vi "Drive Train Global.vi"() -> ()   [LabVIEW 2018]
panel:
  in  "Robot Stopped?":bool=TRUE
  in  "Reset Field Position":bool
  in  "Wheel Angle Offsets Practice Bot":T1={"FrontLeft"=-142.0, "FrontRight"=107.85, "BackLeft"=-87.1, "BackRight"=69.4}
  in  "Angle Locking to":dbl=630.0
  in  "Angle to Lock To":dbl=270.0
  out "Lock to Angle":bool
  out "Robot Centric":bool
  in  "Don't Turn While Translate PID Gains":T2 {"derivative time (Td, min)" format="%.3f"; "integral time (Ti, min)" format="%.3f"; "proportional gain (Kc)" format="%.3f"}
  in  "Zero Yaw":bool
  in  "Wheel Angle Offsets":T1={"FrontLeft"=135.0, "FrontRight"=-169.4, "BackLeft"=-64.0, "BackRight"=-40.1}
  out "Wheel Angles":T1={"FrontLeft"=-0.07255429144282743, "FrontRight"=0.13487537853610831, "BackLeft"=-0.06803657905170724, "BackRight"=-0.04791306754956537}
  in  "Rot. Point Y":dbl
  in  "Rot. Point X":dbl
  in  "Wheel Turn PID Values":T3={"Front Left"={"P Value"=0.014, "I Value"=0.0, "D Value"=0.0}, "Front Right"={"P Value"=0.014, "I Value"=0.0, "D Value"=0.0}, "Back Left"={"P Value"=0.014, "I Value"=0.0, "D Value"=0.0}, "Back Right"={"P Value"=0.014, "I Value"=0.0, "D Value"=0.0}}
  in  "Z Command":dbl
  in  "Y Command":dbl=-0.0
  out "Gyro Information":T4={"Rollover"=0.0, "Yaw"=-1.63, "Cont Yaw"=-1.63}
  in  "X Command":dbl=-0.01165823673846645
  in  "Current State":enum16{"Reached Position", "Going to Position"}(ring)
  in  "Current Mode":T5(ring)=enum."Field Oriented"
  out "Extra Info":bool
  out "Velocity":cluster{"X":dbl, "Y":dbl}
  out "Position":cluster{"X":dbl, "Y":dbl}={"X"=0.31095361119092635, "Y"=-0.2016841928455702}
  out "Wheel Drive Encoders":cluster{"Rates":dbl[], "Distances":dbl[]}={"Rates"=[0.0, 0.0, 0.0, -0.0], "Distances"=[0.9954750000000001, -0.01917175, -0.287145, -0.0]}
  # "X Command is spin"
  # "Z is X"
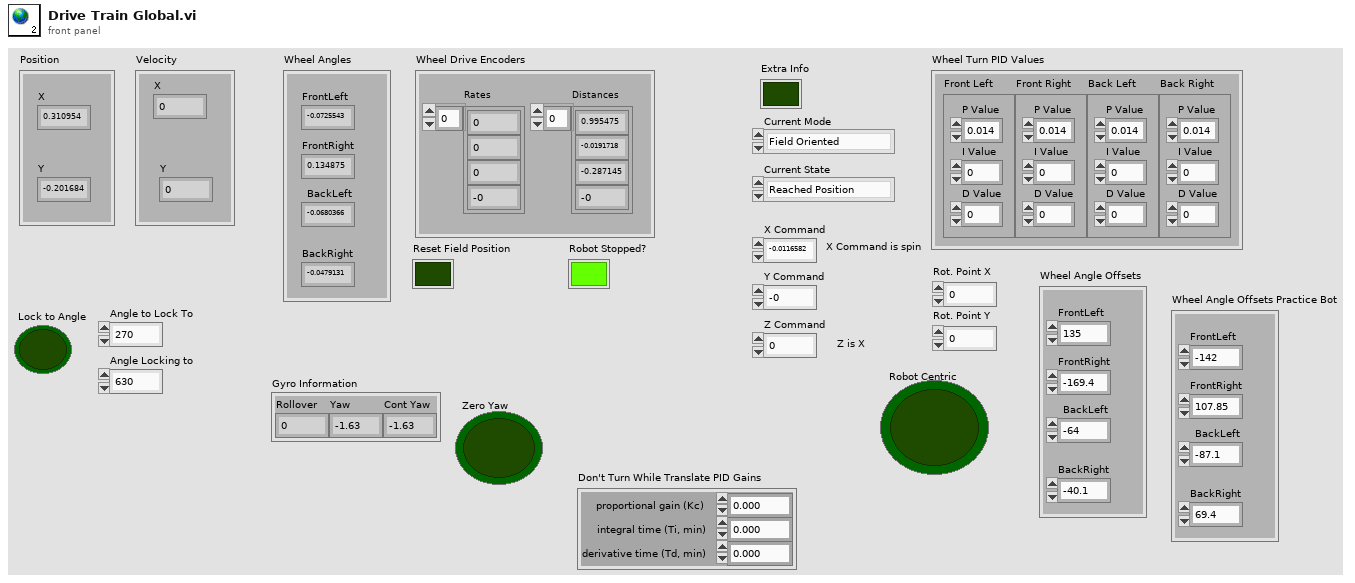
[diagram p1: front panel]
types:
  T1 = cluster{"FrontLeft":dbl, "FrontRight":dbl, "BackLeft":dbl, "BackRight":dbl}
  T2 = cluster{"proportional gain (Kc)":dbl, "integral time (Ti, min)":dbl, "derivative time (Td, min)":dbl}
  T3 = cluster{"Front Left":cluster{"P Value":dbl, "I Value":dbl, "D Value":dbl}, "Front Right":cluster{"P Value":dbl, "I Value":dbl, "D Value":dbl}, "Back Left":cluster{"P Value":dbl, "I Value":dbl, "D Value":dbl}, "Back Right":cluster{"P Value":dbl, "I Value":dbl, "D Value":dbl}}
  T4 = cluster{"Rollover":dbl, "Yaw":dbl, "Cont Yaw":dbl}
  T5 = enum16{"Autonomous Mode", "Field Oriented", "Robot Oriented", "Tank Mode"}
diagram:
